vi "HEWH End Of Test Display.vi"(7 "String Notifier":string="MessageA", 8 "error in (no error)":errorcluster, 10 "Disable Station":bool, 11 "Current Cond":T1) -> (0 "error out":errorcluster, 3 "Failure":bool)   [LabVIEW 2023]
uses:
  Draw Water Specific/Type Definitions/HEWH Special Condition Check.ctl
  Utility/Type Definitions/UTILITY Notifier.ctl
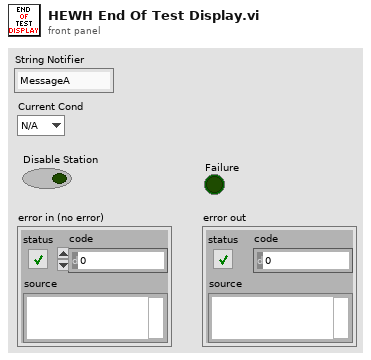
[diagram p1: front panel]
types:
  T1 = typedef "HEWH Special Condition Check.ctl" = enum16{"N/A", "C1", "C2", "Reset/Fail", "Skip Draw Sequence"}
  T2 = typedef "UTILITY Notifier.ctl" = enum16{"Set", "Read", "Release Ref"}
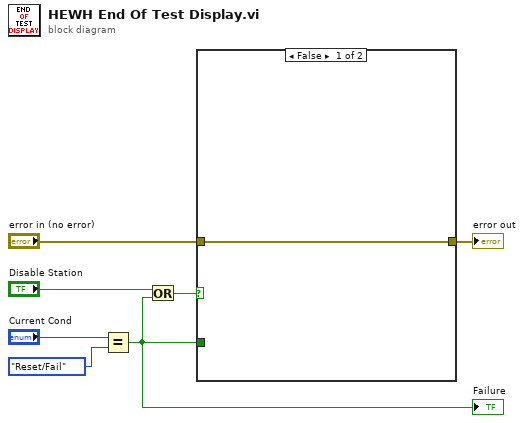
[diagram p0: block diagram]
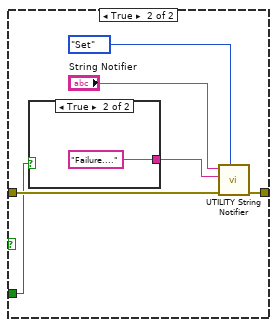
[diagram p2: hidden frame]
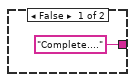
[diagram p3: hidden frame]
diagram:
  n1 = Equal?(x="Current Cond", y=HEWH_Special_Condition_Check."Reset/Fail") -> (x = y?=w7:bool)
  "Failure" <- w7
  n2 = Or(x="Disable Station", y=w7) -> (x .or. y?=w6:bool)
  n3 = case shown="False" w6 {
    tunnel: "error in (no error)" -> [w8 w13]
    tunnel: [w8 w12] -> w2
    tunnel: w7 -> [_ w9]
    frame False {
    }
    frame True {
      n4 = case shown="True" w9 {
        tunnel: ["Complete...." ("Set Status") "Failure...." ("Set Status")] -> w11
        frame False {
        }
        frame True {
        }
      }
      n5 = call "UTILITY String Notifier.vi"("Status"=UTILITY_Notifier."Set", "error in (no error)"=w13, "Set Status"=w11, "name (unnamed)"="String Notifier") -> ("error out"=w12:errorcluster)  [unwired: 6 in, 1 out]
    }
  }
  "error out" <- w2
